vi "Get String Data Size.vi"(10 "Data String":u8[](array[numeric])) -> (2 "Data Size":i32)   [LabVIEW 2017, in "Composition.lvlib"]
doc: "Gets the data size of a string"
uses:
  Composition.lvlib
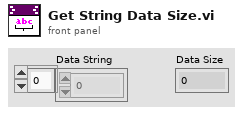
[diagram p1: front panel]
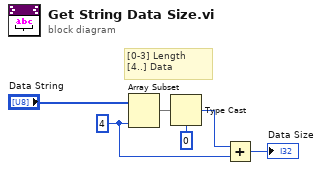
[diagram p0: block diagram]
diagram:
  w3 = 4 ("length")
  # "[0-3] Length\n[4..] Data"
  n1 = Array Subset(array="Data String", length=w3) -> (w4:u8[])  [unwired: 1 in]
  n2 = Type Cast(type=0, x=w4) -> (*(type *) &x=w5:i32)
  n3 = Add(x=w5, y=w3) -> (x+y=→"Data Size":i32)
